vi "Log Message.vi"(8 "error in (no error)":errorcluster, 10 "Log Message":string, 11 "Controller in":refnum<class "Controller.lvclass">) -> (0 "error out":errorcluster, 3 "Controller out":refnum<class "Controller.lvclass">)   [LabVIEW 2021, in "Controller.lvlib" / "Controller.lvclass"]
uses:
  Controller.lvclass
  UserInterface/UserInterface Messages/Log Data Msg/Log Data Msg.lvclass
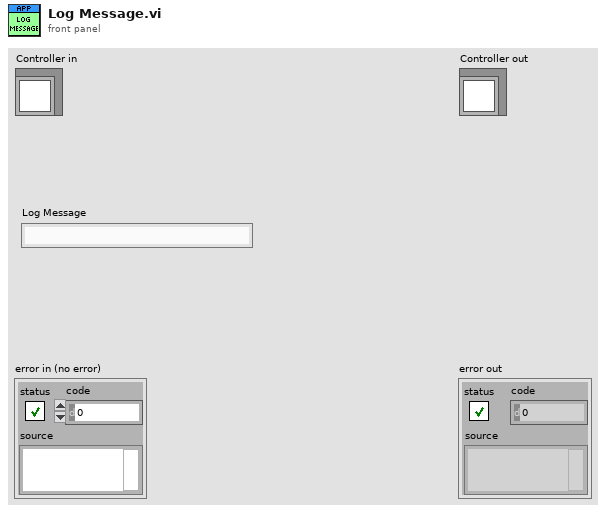
[diagram p1: front panel]
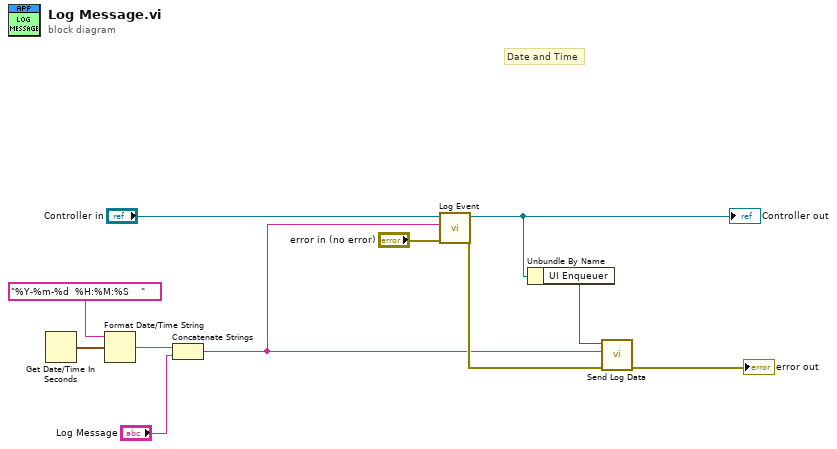
[diagram p0: block diagram]
diagram:
  # "Date and Time"
  n1 = Get Date/Time In Seconds() -> (seconds since 1Jan1904=w4:timestamp)
  n2 = Format Date/Time String(time format string (%c)="%Y-%m-%d  %H:%M:%S    ", seconds (now)=w4) -> (date/time string=w3:string)  [unwired: 1 in]
  n3 = Concatenate Strings(w3, "Log Message") -> (w6:string)
  n4 = call-dynamic "Log Event.vi"("error in (no error)"="error in (no error)", "String"=w6, "Controller in"="Controller in") -> ("error out"=w8:errorcluster, "Controller out"=w1:refnum<class "Controller.lvclass">)  [unwired: 7 in]
  "Controller out" <- w1
  n5 = Unbundle By Name(w1) -> ("UI Enqueuer"=w10:refnum<class "Message Enqueuer.lvclass">)
  n6 = call "Send Log Data.vi"("error in (no error)"=w8, "Message"=w6, "Message Enqueuer"=w10) -> ("error out"=→"error out":errorcluster)  [unwired: 7 in, 1 out]
